vi "DisplayMenuItemSelected.vi"(4 "Occurrence Refnum":refnum<k4>, 5 "Menu Items":T1(array[cluster]), 6 "Menu Refnum":refnum<k9>) -> ()   [LabVIEW 2011]
panel:
  out "error out":errorcluster
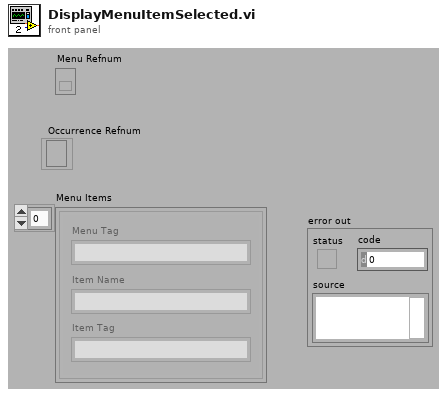
[diagram p1: front panel]
types:
  T1 = cluster{"Menu Tag":string, "Item Name":string, "Item Tag":string}[]
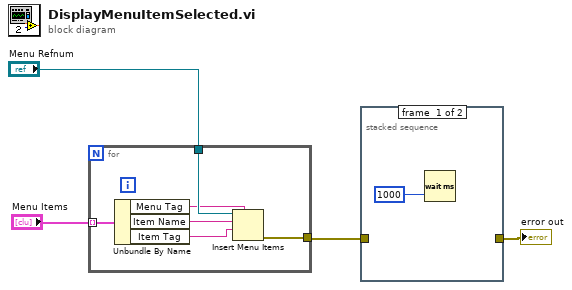
[diagram p0: block diagram]
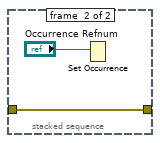
[diagram p2: hidden frame]
diagram:
  n1 = for {
    tunnel: "Menu Refnum" -> [w10]
    tunnel: "Menu Items" -> [w9] mode=indexing
    tunnel: [w7] -> w1
    n2 = Unbundle By Name(w9) -> ("Menu Tag"=w5:string, "Item Name"=w8:string, "Item Tag"=w6:string)
    n3 = Insert Menu Items(5:w5, 7:w6, 8:w8, 9:w10) -> (0:w7:errorcluster)  [unwired: 1 in, 3 out]
  }
  n4 = stacked-sequence {
    tunnel: [_ w13] -> w2
    tunnel: w1 -> [_ w13]
    frame #0 {
      n5 = Wait (ms)(milliseconds to wait=u32 1000) -> ()  [unwired: 1 out]
    }
    frame #1 {
      n6 = Set Occurrence("Occurrence Refnum") -> ()
    }
  }
  "error out" <- w2
